vi "TCP Wait For Specific Response.vi"(0 "TCP Connection In":refnum<k5>, 1 "Next response (t)":bool=TRUE, 5 "Expected Type":T3=enum."NONE", 7 "Expected Subtype (none)":T1, 9 "Expected Message Start (\"\":any)":string, 11 "error in":errorcluster, 12 "Timeout (250 ms)":i32=250) -> (4 "TCP Connection Out":refnum<k5>, 6 "TCP Messages":string[](array[string]), 8 "Desired Response":T2, 15 "error out":errorcluster)   [LabVIEW 2012]
uses:
  Controls/QCA NART Response Type.ctl
  Controls/QCA NART Message.ctl
  Controls/QCA NART Response SubType.ctl
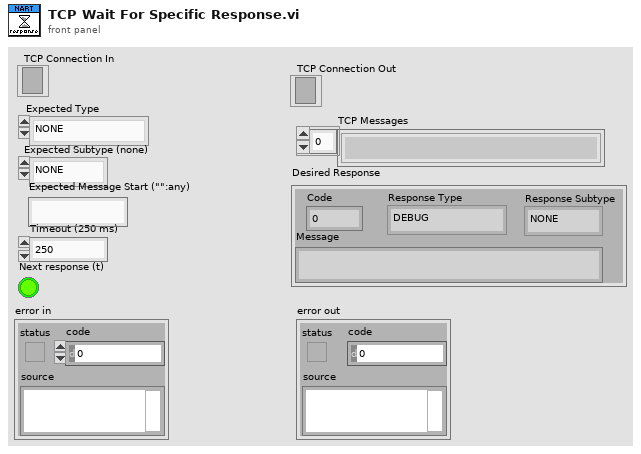
[diagram p1: front panel]
types:
  T1 = typedef "QCA NART Response SubType.ctl" = enum16{"NONE", "OK", "ON", "OFF", "BEGIN", "DONE"}
  T2 = typedef "QCA NART Message.ctl" = cluster{"Code":dbl, "Response Type":T3, "Response Subtype":T1, "Message":string}
  T3 = typedef "QCA NART Response Type.ctl" = enum16{"DEBUG", "CONTROL", "INFO", "WARNING", "ERROR", "NONE"}
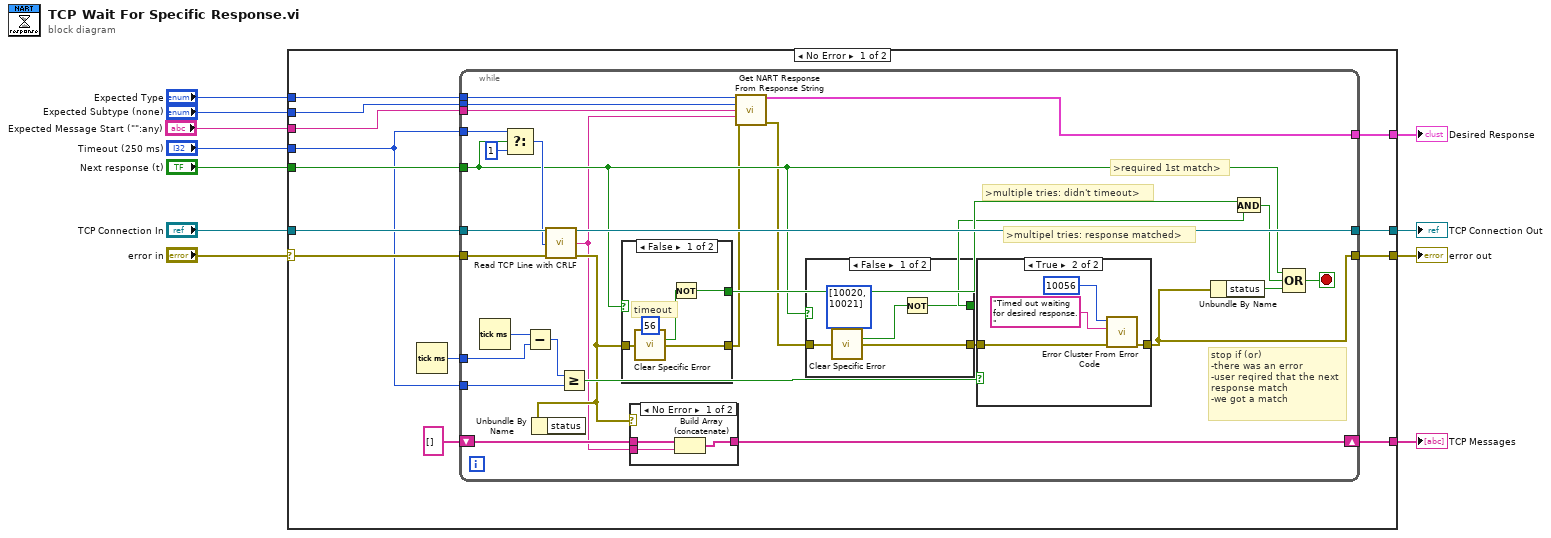
[diagram p0: block diagram]
diagram:
  n1 = case shown="No Error" "error in" {
    selector: "error in" -> [w24 w76]
    tunnel: [w15 w76] -> w8
    tunnel: "TCP Connection In" -> [w23 w75]
    tunnel: [w22 w75] -> w10
    tunnel: "Timeout (250 ms)" -> [w16 _]
    tunnel: [w19 _] -> w6
    tunnel: "Expected Type" -> [w21 _]
    tunnel: "Expected Subtype (none)" -> [w20 _]
    tunnel: "Next response (t)" -> [w18 _]
    tunnel: [w14 _] -> w2
    tunnel: "Expected Message Start (\"\":any)" -> [w12 _]
    frame No Error {
      n2 = Tick Count (ms)() -> (millisecond timer value=w17:u32)
      n3 = while {
        tunnel: w24 -> [w53]
        tunnel: w23 -> [w52]
        tunnel: [w51] -> w22
        tunnel: w21 -> [w27]
        tunnel: w20 -> [w28]
        tunnel: [w30] -> w19
        tunnel: w16 -> [w37]
        tunnel: w18 -> [w36]
        tunnel: w17 -> [w48]
        tunnel: w16 -> [w46]
        tunnel: [w42] -> w15
        shift-right: [w34] -> w14
        shift-left: string[] [] -> [w33]
        tunnel: w12 -> [w29]
        stop <- w43 stop-if-true
        # ">required 1st match>"
        # ">multipel tries: response matched>"
        # ">multiple tries: didn't timeout>"
        # "stop if (or)\n-there was an error\n-user reqired that the next response match\n-we got a match"
        n4 = Tick Count (ms)() -> (millisecond timer value=w49:u32)
        n5 = Select(t=w37, s=w36, f=1) -> (s? t:f=w50:i32)
        n6 = Subtract(x=w49, y=w48) -> (x-y=w47:u32)
        n7 = call "Read TCP Line with CRLF.vi"("TCP Connection In"=w52, "timeout ms (100)"=w50, "error in"=w53) -> ("TCP Connection Out"=w51:refnum<k5>, "TCP Line"=w25:string, "error out"=w26:errorcluster)  [unwired: 10 in]
        n8 = Unbundle By Name(w26) -> ()  [unwired: 1 out]
        n9 = Greater Or Equal?(x=w47, y=w46) -> (x >= y?=w45:bool)
        n10 = case shown="False" w36 {
          tunnel: w26 -> [w68 w69]
          tunnel: [w67 w69] -> w32
          tunnel: [w64 _] -> w40
          frame False {
            # "timeout"
            n11 = call "Clear Specific Error.vi"("Specific Error Number (0: none)"=56 ("Specific Error Number"), "error in"=w68) -> ("Error Cleared?"=w65:bool, "error out"=w67:errorcluster)  [unwired: 12 in]
            n12 = Not(x=w65) -> (.not. x?=w64:bool)
          }
          frame True {
            # "1 try"
          }
        }
        n13 = case shown="No Error" w26 {
          tunnel: [w56 w57] -> w34
          tunnel: w33 -> [w55 w57]
          tunnel: w25 -> [w54 _]
          frame No Error {
            n14 = Build Array (concatenate)(w55, w54) -> (w56:string[])
          }
          frame Error {
          }
        }
        n15 = call "Get NART Response From Response String.vi"("Expected Response"=w27, "Response Subtype"=w28, "Expected Message start (\"\":any)"=w29, "TCP Line"=w25, "error in (no error)"=w32) -> ("NART Message"=w30:T2, "error out"=w31:errorcluster)  [unwired: 9 in]
        n16 = case shown="False" w36 {
          tunnel: w31 -> [w62 w63]
          tunnel: [w61 w63] -> w41
          tunnel: [w59 _] -> w39
          frame False {
            n17 = call "Clear Specific Error.vi"("Error Numbers Array (emtpy)"=i32[] [10020, 10021] ("Error Numbers Array"), "error in"=w62) -> ("Error Cleared?"=w60:bool, "error out"=w61:errorcluster)  [unwired: 12 in]
            n18 = Not(x=w60) -> (.not. x?=w59:bool)
          }
          frame True {
            # "1 try"
          }
        }
        n19 = case shown="True" w45 {
          tunnel: w41 -> [w70 w74]
          tunnel: [w70 w72] -> w42
          frame False {
          }
          frame True {
            n20 = call <vilib>:"Error Cluster From Error Code.vi"("error in (no error)"=w74, "error message (\"\")"="Timed out waiting for desired response." ("format string"), "error code (0)"=10056) -> ("error out"=w72:errorcluster)  [unwired: 6 in]
          }
        }
        n21 = Unbundle By Name(w42) -> ("status"=w44:bool)
        n22 = And(x=w40, y=w39) -> (x .and. y?=w38:bool)
        n23 = Compound Arithmetic op=OR(w36, w38, w44) -> (w43:bool)
      }
    }
    frame Error {
    }
  }
  "TCP Connection Out" <- w10
  "error out" <- w8
  "Desired Response" <- w6
  "TCP Messages" <- w2
